vi "Get Element Types.vi"(8 "error in (no error)":errorcluster, 11 "JSON Array in":refnum<class "JSON Array.lvclass">) -> (0 "error out":errorcluster, 1 "single type?":bool, 2 "types":T1[](array[typedef]), 3 "JSON Array out":refnum<class "JSON Array.lvclass">)   [LabVIEW 2017, in "LVJSON.lvlib" / "JSON Array.lvclass"]
uses:
  JSON Array.lvclass
  JSON Types.ctl
  JSON Array.lvclass/JSON Array.ctl
  JSON Datatype/JSON Datatype.lvclass
  LVJSON.lvlib
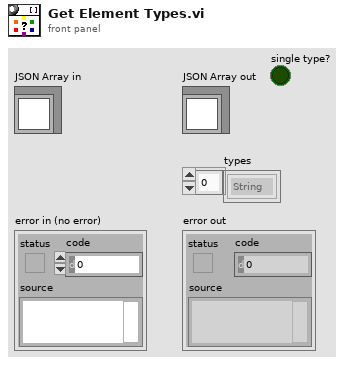
[diagram p1: front panel]
types:
  T1 = typedef "LVJSON.lvlib/JSON Types.ctl" = enum16{"String", "Numeric", "Boolean", "NULL", "Object", "1D Array", "Unknown"}
  T2 = typedef "JSON Types.ctl" = enum16{"String", "Numeric", "Boolean", "NULL", "Object", "1D Array", "Unknown"}
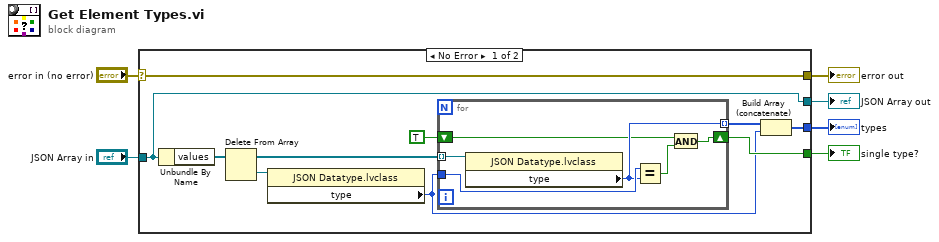
[diagram p0: block diagram]
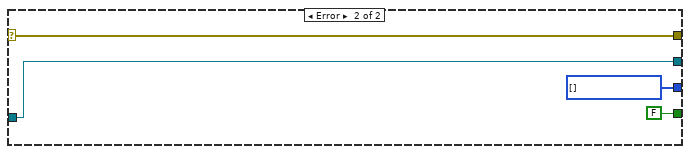
[diagram p2: hidden frame]
diagram:
  n1 = case shown="No Error" "error in (no error)" {
    selector: "error in (no error)" -> [w16 w26]
    tunnel: [w16 w26] -> w5
    tunnel: [w15 w25] -> w3
    tunnel: "JSON Array in" -> [w15 w25]
    tunnel: [w8 w24] -> w2
    tunnel: [w10 FALSE] -> w1
    frame No Error {
      n2 = Unbundle By Name(w15) -> ("values"=w14:refnum<class "JSON Datatype.lvclass">[])
      n3 = Delete From Array(array=w14) -> (deleted portion=w13:refnum<class "JSON Datatype.lvclass">, array with subset deleted=w12:refnum<class "JSON Datatype.lvclass">[])  [unwired: 2 in]
      n4 = property class="JSON Datatype.lvclass"(reference=w13) -> ("type"=w7:T2)  [unwired: 1 in, 2 out]
      n5 = for {
        tunnel: w12 -> [w22] mode=indexing
        tunnel: [w20] -> w9 mode=indexing
        tunnel: w7 -> [w21]
        shift-right: [w17] -> w10
        shift-left: TRUE -> [w18]
        n6 = property class="JSON Datatype.lvclass"(reference=w22) -> ("type"=w20:T2)  [unwired: 1 in, 2 out]
        n7 = Equal?(x=w21, y=w20) -> (x = y?=w19:bool)
        n8 = And(x=w18, y=w19) -> (x .and. y?=w17:bool)
      }
      n9 = Build Array (concatenate)(w9, w7) -> (w8:T2[])
    }
    frame Error {
      w24 = T1[] [] items=["String", "Numeric", "Boolean", "NULL", "Object", "1D Array", "Unknown"]
    }
  }
  "error out" <- w5
  "JSON Array out" <- w3
  "types" <- w2
  "single type?" <- w1
